vi "3D_Traverse_move.vi"(0 "Mode":T5=enum."Read traverse position", 1 "Position":sgl[](array[numeric])=[0.0, 0.0, 0.0] format="%#.2f", 2 "Extra command String":string, 3 "Work in Tunnel Coordinates":T3, 4 "Home":T2, 5 "Simulate/Run":T4=enum."Run VI", 6 "Route Checking?":bool=TRUE, 7 "Traverse name":string, 8 "Display Error":bool=TRUE, 9 "Backlash Compensation?":bool=TRUE, 10 "Row Number":i32=-1, 11 "Last Part of Move?":bool=TRUE, 13 "Currently on Point":i32=-1) -> (12 "Model:    Roll        Pitch         Yaw  (deg)":sgl[](array[numeric]) caption="ModelRollPitchYaw (deg)" format="%#.2f", 14 "Trav Position achieved":sgl[](array[numeric]) format="%#.2f", 17 "Valid Steps before Trav to Trav (Tun Cord)":sgl[][](array[numeric]), 19 "Error String":string)   [LabVIEW 2022 SP3]
uses:
  Trav_mode.ctl
  Controls/User_Specific_mode.ctl
  Controls/Tunnel_Coordinates.ctl
  Controls/Home.ctl
  Controls/Position Feedback System.ctl
  Route mapping/Route_Display_Mode.ctl
  ADAM Client/Sub VIs/ADAM Controls/Quick_local_ADAM_Table.ctl
  Controls/In_Range.ctl
  Globals/Trav_pos_global.vi
  Globals/Preference_global.vi
  Globals/Constants_global.vi
  Route mapping/Route_mapping_global.vi
  Globals/Extra_Commands_Global.vi
panel:
  out "Position Feedback System":T1
  out "Feedback Correction":sgl[](array[numeric]) format="%#.2f"
  out "Start Position":sgl[](array[numeric])
  out "Move Time (s)":sgl
  in  "Position Offset":sgl[](array[numeric])=[0.0, 0.0, 0.0] step=1 format="%#.2f"
  out "Traverses Available":string[](array[string])
  in  "Traverse":u16(ring) items=["A_Tunnel", "A_Tunnel_Turntable", "Pitch_Yaw", "Pitch_Traverse", "Dynamixel_Pitch"]
  # "X                Y                   Z"
  # "X                Y                   Z"
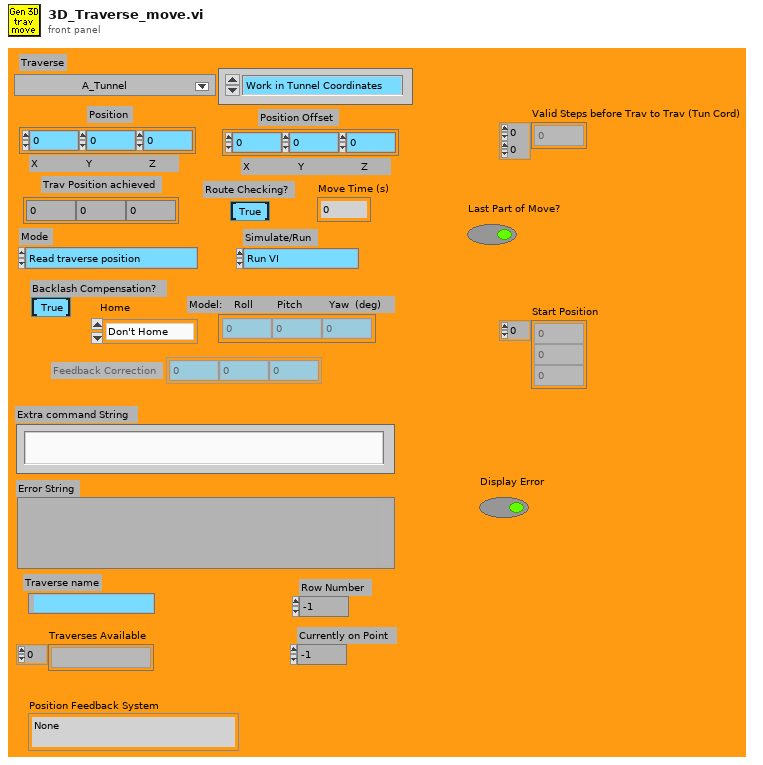
[diagram p1: front panel]
types:
  T1 = typedef "Position Feedback System.ctl" = enum16{"None", "OptiTrack"}
  T2 = typedef "Home.ctl" = enum16{"Don't Home", "Home  +X", "Home  -X", "Home  +Y", "Home  -Y", "Home  +Z", "Home  -Z"}
  T3 = typedef "Tunnel_Coordinates.ctl" = enum16{"Work in Tunnel Coordinates", "Work in Model Coordinates"}
  T4 = typedef "User_Specific_mode.ctl" = enum16{"Check VI only", "Run VI"}
  T5 = typedef "Trav_mode.ctl" = enum16{"Move traverse", "Read traverse position", "Teach Position"}
  T6 = enum8{"Enabled", "Disabled", "Disabled and Grayed Out"}
  T7 = enum16{"To Traverse Coordinates", "To User Coordinates"}
  T8 = typedef "Route_Display_Mode.ctl" = enum16{"Display View Always", "Display View on Crash"}
  T9 = typedef "Quick_local_ADAM_Table.ctl" = enum16{"Read Global", "Load Global From ADAM Table", "Write Global"}
  T10 = typedef "In_Range.ctl" = enum16{"%", "±", "% & ±"}
  T11 = typedef "Traverse_cluster.ctl" = cluster{"Start X":sgl, "Start Y":sgl, "Start Z":sgl, "End X":sgl, "End Y":sgl, "End Z":sgl, "nPoints":i32, "Spacing":T12, "Filename":path, "Tunnel Speed":dbl, "Averaging time (mins)":dbl, "Extra Commands":string, "Carrier_1 Q (l/min)":dbl, "Carrier_2 Q (l/min)":dbl, "Trace Gas Concentration (%)":dbl, "Specific Arguments":string, "Comments":string, "Row No":i32, "Row Type Selector":T13, "EstCompl":string, "Row Duration (mins)":dbl, "nValidPoints":i32, "Meas Setup File":string}
  T12 = typedef "Spacing.ctl" = enum16{"Linear", "Log", "Gauss", "Specified", "N/A"}
  T13 = typedef "Multi_run_mode.ctl" = enum16{"Move Traverse Only", "Set Tunnel Speed Only", "Set Source Only", "Set Measurement Conditions", "Single Measurement", "Vertical Profile", "Lateral Profile", "Longitudinal Profile", "Multi-Axis Profile", "Explore Volume", "Auto Calibrate", "Meas Fast FID Bkgnd", "Check Beam Power", "Scanning Valve Measurement", "Run VI Named:", "Set ADAM Ch", "Wait (minutes)", "Send Message", "Synchronize With:", "Fall Back to this Row", "Turn Off Row Repeating", "Traverse 3D Volume", "Blank Row", "Jump to Fall Back Row"}
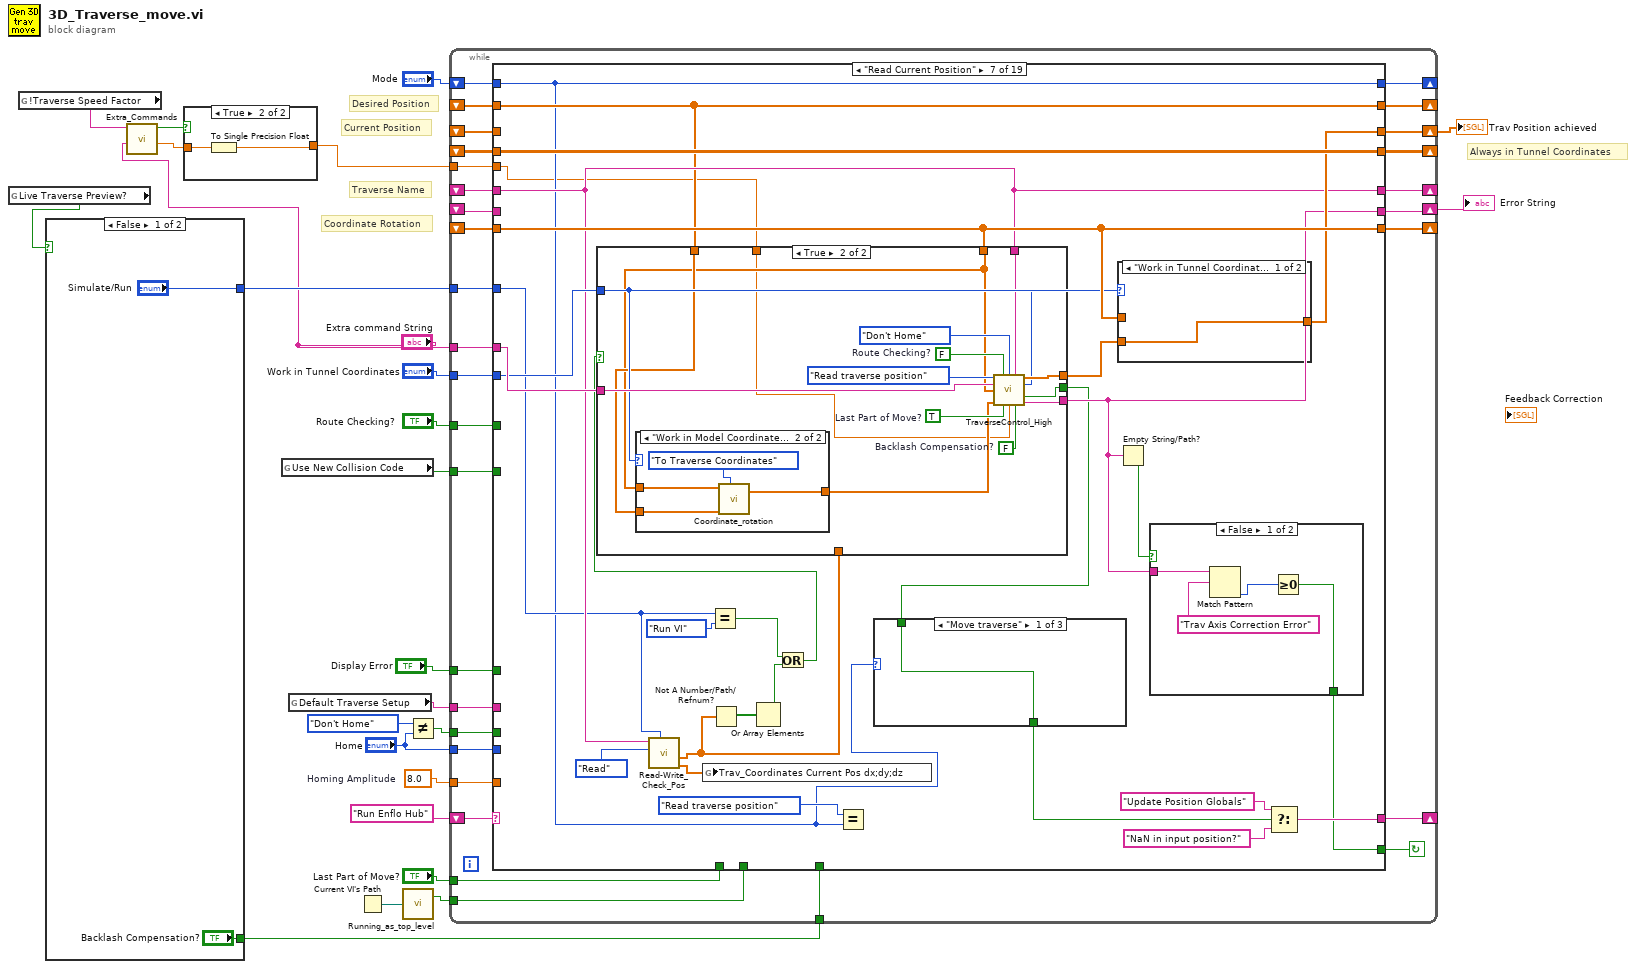
[diagram p0: block diagram]
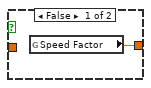
[diagram p2: hidden frame]
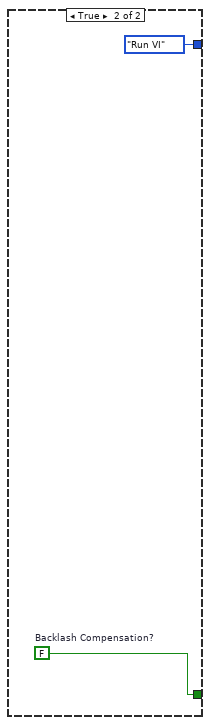
[diagram p3: hidden frame]
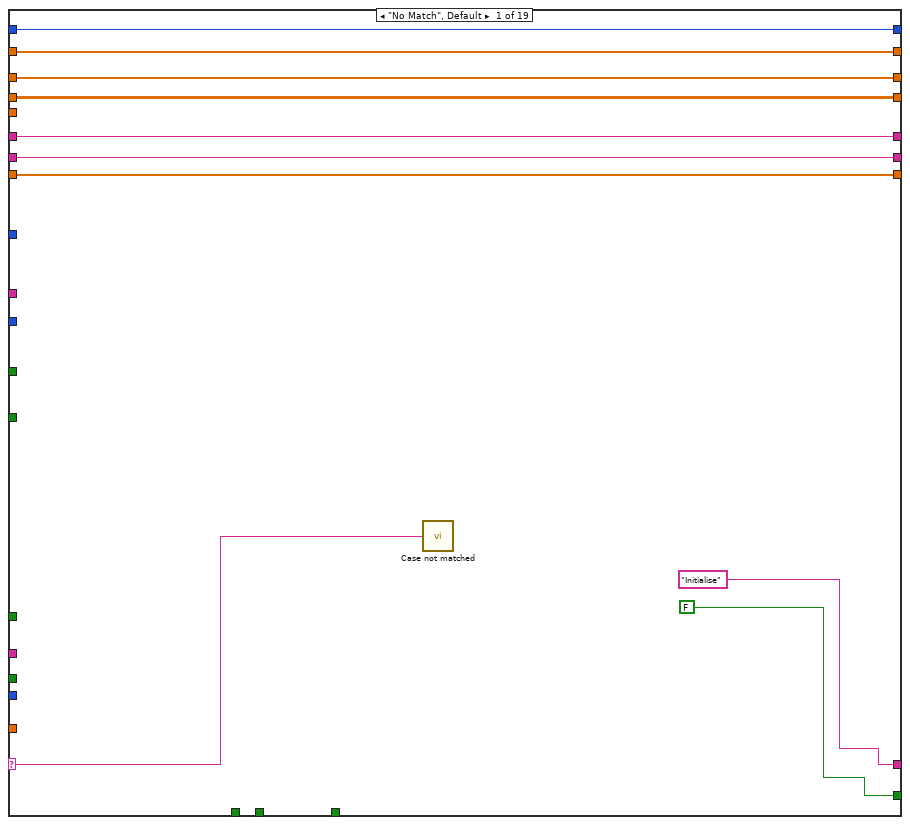
[diagram p4: hidden frame]
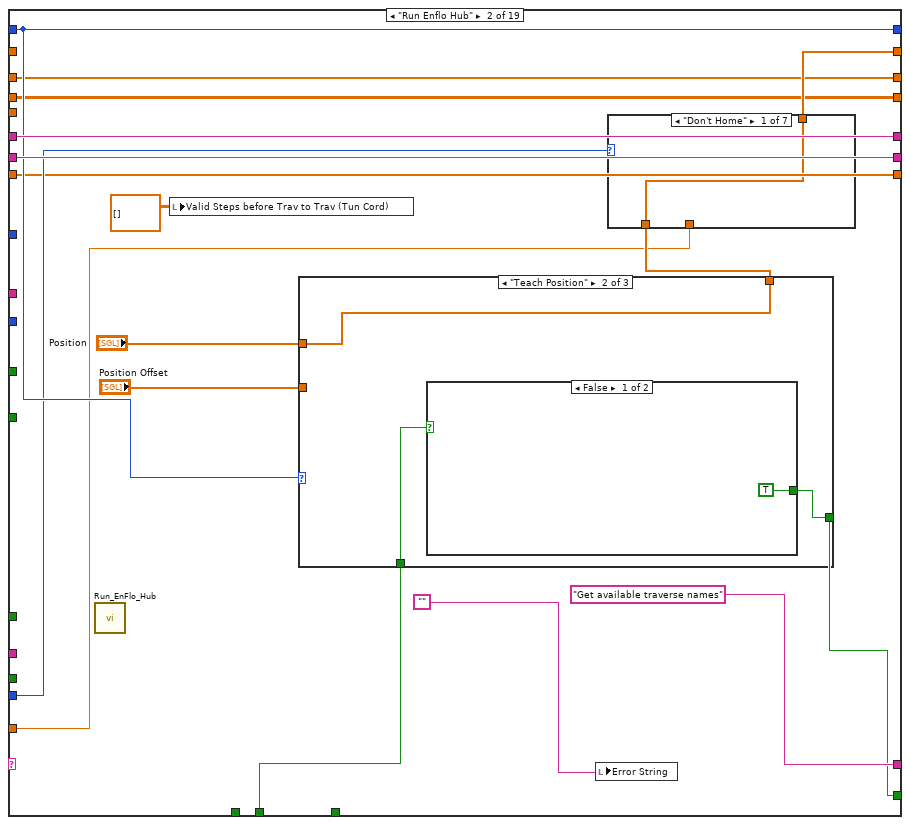
[diagram p5: hidden frame]
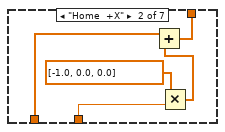
[diagram p6: hidden frame]
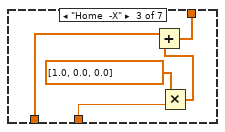
[diagram p7: hidden frame]
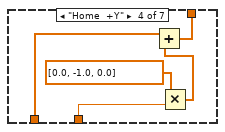
[diagram p8: hidden frame]
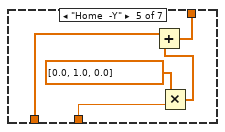
[diagram p9: hidden frame]
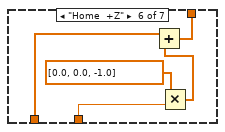
[diagram p10: hidden frame]
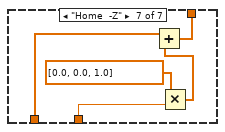
[diagram p11: hidden frame]
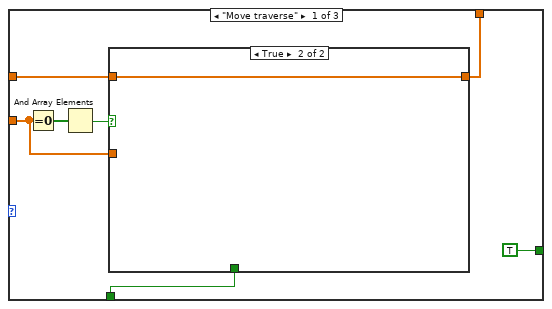
[diagram p12: hidden frame]
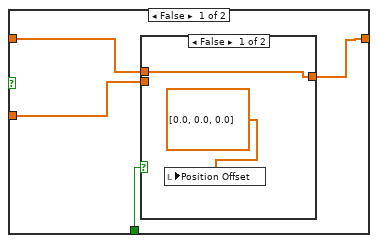
[diagram p13: hidden frame]
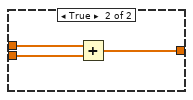
[diagram p14: hidden frame]
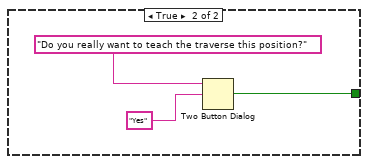
[diagram p15: hidden frame]
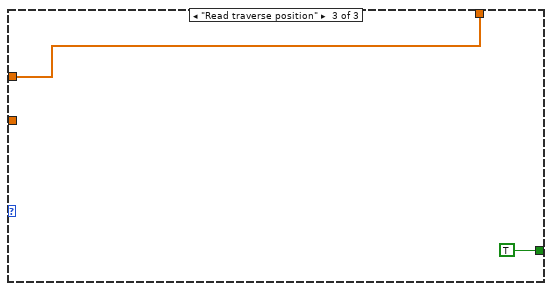
[diagram p16: hidden frame]
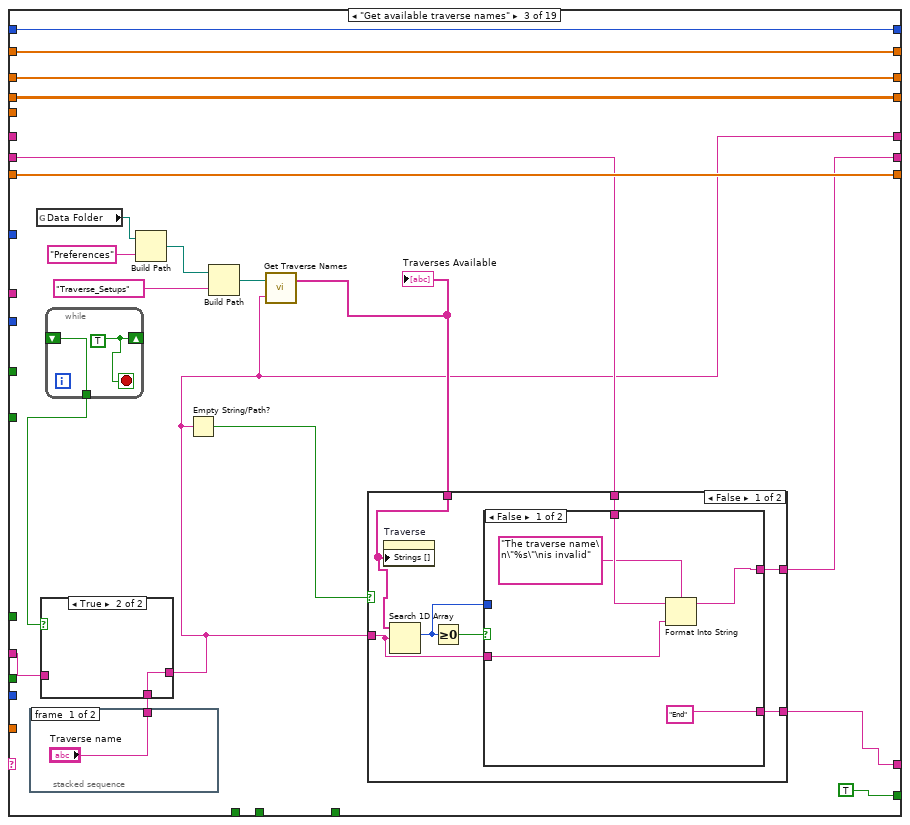
[diagram p17: hidden frame]
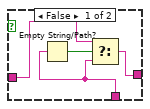
[diagram p18: hidden frame]
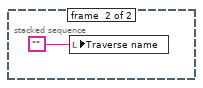
[diagram p19: hidden frame]
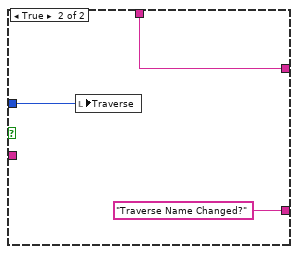
[diagram p20: hidden frame]
diagram:
  w16 = sgl 8.0  # Homing Amplitude
  # "Desired Position"
  # "Always in Tunnel Coordinates"
  # "Current Position"
  # "Coordinate Rotation"
  # "Traverse Name"
  n1 = global read "Trav_pos_global.vi" "Live Traverse Preview?"() -> (w6:bool)
  n2 = global read "Extra_Commands_Global.vi" "!Traverse Speed Factor"() -> (w5:string)
  n3 = case shown="False" w6 {
    tunnel: ["Simulate/Run" User_Specific_mode."Run VI" ("Simulate/Run")] -> w23
    tunnel: ["Backlash Compensation?" w27] -> w7
    frame False {
    }
    frame True {
      w27 = FALSE  # Backlash Compensation?
    }
  }
  n4 = call "Extra_Commands.vi"("String to Search"="Extra command String", "Command"=w5) -> ("Numeric Value"=w4:dbl, "Command Found"=w3:bool)  [unwired: 1 in, 3 out]
  n5 = case shown="True" w3 {
    tunnel: w4 -> [_ w31]
    tunnel: [w29 w30] -> w1
    frame False {
      n6 = global read "Trav_pos_global.vi" "Speed Factor"() -> (w29:sgl)
    }
    frame True {
      n7 = To Single Precision Float(number=w31) -> (single precision float=w30:sgl)
    }
  }
  n8 = global read "Preference_global.vi" "Use New Collision Code"() -> (w12:bool)
  n9 = global read "Trav_pos_global.vi" "Default Traverse Setup"() -> (w18:string)
  n10 = Current VI's Path() -> (path=w10:path)
  n11 = call "Running_as_top_level.vi"("Vi path name"=w10) -> ("Top Level"=w9:bool)  [unwired: 1 out]
  n12 = Not Equal?(x=Home."Don't Home" ("Home"), y="Home") -> (x != y?=w13:bool)
  n13 = while {
    shift-left: "Run Enflo Hub" -> [w60]
    shift-right: [w61] -> _
    shift-right: [w58] -> _
    shift-left: _ -> [w34]
    tunnel: w23 -> [w59]
    shift-right: [w57] -> w22
    shift-left: _ -> [w56]
    shift-right: [w54] -> _
    shift-left: _ -> [w55]
    shift-right: [w51] -> _
    shift-left: _ -> [w50]
    shift-right: [w52] -> w19
    shift-left: _ -> [w53]
    tunnel: "Work in Tunnel Coordinates" -> [w49]
    tunnel: "Route Checking?" -> [w48]
    tunnel: w18 -> [w47]
    shift-right: [w46] -> _
    shift-left: _ -> [w45]
    shift-right: [w43] -> _
    shift-left: "Mode" -> [w44]
    tunnel: "Home" -> [w42]
    tunnel: w16 -> [w41]
    tunnel: w13 -> [w40]
    tunnel: w12 -> [w39]
    tunnel: "Last Part of Move?" -> [w38]
    tunnel: w9 -> [w37]
    tunnel: "Extra command String" -> [w36]
    tunnel: "Display Error" -> [w35]
    tunnel: w7 -> [w33]
    tunnel: w1 -> [w32]
    stop <- w62 continue-if-true
    n14 = case shown="\"Read Current Position\"" w60 {
      selector: w60 -> [w63 _ _ _ _ _ _ _ _ _ _ _ _ _ _ _ _ _ _]
      tunnel: [FALSE w85 TRUE TRUE w220 TRUE w307 TRUE ("T button?") w400 w526 w636 TRUE ("Display Trav 2 Trav Error") TRUE ("Display Trav 2 Trav Error") TRUE ("Display Trav 2 Trav Error") TRUE ("Display Trav 2 Trav Error") TRUE TRUE TRUE FALSE] -> w62
      tunnel: ["Initialise" "Get available traverse names" w158 "Traverse Name Changed?" "Mode" w260 w312 w358 w401 w527 w637 w666 "End" w721 "Update Position Globals" "Update Position Globals" "Tidy up" "End" "End"] -> w61
      tunnel: w59 -> [_ _ _ _ w214 w261 w296 _ w412 w537 w640 _ _ w732 _ _ w856 w898 w989]
      tunnel: [w70 w88 w147 w193 w226 w257 w304 w369 w404 w530 w634 w677 w705 w738 w765 w800 w855 w903 w993] -> w58
      tunnel: [w69 w87 w157 w205 w221 w262 w308 w366 w394 w539 w630 w661 w710 w735 w777 w787 w859 w905 w995] -> w57
      tunnel: w34 -> [w70 w88 _ _ w226 w257 w304 w369 w404 w530 w634 w677 w705 w738 w765 w800 w855 w903 w993]
      tunnel: w56 -> [w69 w87 w156 w205 _ w262 _ w366 _ _ w625 w673 w710 w735 w777 _ w859 w906 w994]
      tunnel: w55 -> [w68 w76 w166 w204 _ w254 w317 w356 w405 w531 w633 w669 w708 w741 w771 w799 w852 w908 w999]
      tunnel: [w68 w76 w166 w204 w225 w254 w317 w356 w405 w531 w633 w669 w708 w741 w771 w799 w852 w908 w999] -> w54
      tunnel: w53 -> [w67 w75 w165 w203 w235 w253 _ w355 w413 w538 w626 w676 w714 w740 w770 _ w854 w907 w1000]
      tunnel: [w67 w75 w165 w203 w235 w253 w311 w355 w413 w538 w628 w676 w714 w740 w770 w797 w854 w907 w1000] -> w52
      tunnel: [w66 w74 w164 w202 w227 w251 w318 w360 w403 w529 w623 w675 w713 w739 w769 w791 w860 w909 w1004] -> w51
      tunnel: w50 -> [w66 w74 w164 w202 w227 w250 w318 w359 _ _ w623 w675 w713 w739 w769 w791 w860 w909 w1004]
      tunnel: w49 -> [_ _ _ _ _ w255 w306 w357 w414 w540 w632 w670 w709 _ w772 w782 w853 _ w1001]
      tunnel: w48 -> [_ _ _ _ _ _ _ w362 _ _ _ _ _ _ _ w795 _ _ _]
      tunnel: w47 -> [_ _ w151 w197 _ _ _ _ _ _ _ _ _ _ _ _ _ _ _]
      tunnel: [w65 w80 w154 w195 w228 w252 w295 w361 w411 w536 w627 w672 w707 w727 w776 w794 w858 w902 w1002] -> w46
      tunnel: w45 -> [w65 _ w154 w195 w228 w252 w295 w363 w411 w536 w627 w672 w707 w727 w776 w794 w858 w902 w1002]
      tunnel: w44 -> [w64 w82 w153 w194 w231 w256 w294 w367 w410 w535 w641 w671 w715 w726 w775 w793 w857 w901 w997]
      tunnel: [w64 w82 w153 w194 w232 w256 w294 w367 w410 w535 w641 w671 w715 w726 w775 w793 w857 w901 w997] -> w43
      tunnel: w42 -> [_ w79 _ _ _ _ _ _ w409 w534 _ _ _ _ _ w788 _ w900 _]
      tunnel: w41 -> [_ w78 _ _ _ _ _ _ w407 w532 _ _ _ _ _ _ _ w899 _]
      tunnel: w40 -> [_ _ _ _ _ _ _ _ _ _ _ _ _ _ _ _ _ w897 _]
      tunnel: w39 -> [_ _ _ _ w229 _ _ _ w406 _ _ w660 _ _ _ _ _ _ _]
      tunnel: w38 -> [_ _ _ _ _ _ _ _ _ _ _ _ _ _ _ w783 _ _ _]
      tunnel: w37 -> [_ w77 _ _ w224 _ _ _ _ _ _ w668 _ _ _ w786 _ _ _]
      tunnel: w36 -> [_ _ _ _ _ _ w310 _ _ _ _ _ _ _ _ w779 _ _ _]
      tunnel: w35 -> [_ _ _ _ _ _ _ _ w399 w525 w635 _ _ _ _ _ _ _ _]
      tunnel: w33 -> [_ _ _ _ _ _ _ _ _ _ _ _ _ _ w766 w780 _ _ _]
      tunnel: w32 -> [_ _ _ _ _ _ w291 _ _ _ _ _ _ _ _ w778 _ _ _]
      frame "No Match", Default {
        n15 = call "Case not matched.vi"("Case Name not Matched"=w63) -> ()
      }
      frame "Run Enflo Hub" {
        n16 = call "Run_EnFlo_Hub.vi"() -> ()  [unwired: 1 in, 7 out]
        n17 = local write "Valid Steps before Trav to Trav (Tun Cord)"(sgl[][] [] ("Valid Steps before Trav to Trav (Tun Cord)")) -> ()
        n18 = case shown="\"Teach Position\"" w82 {
          tunnel: [TRUE ("T button?") w140 TRUE ("T button?")] -> w85
          tunnel: [w124 w139 w146] -> w81
          tunnel: "Position" -> [w123 w139 w146]
          tunnel: "Position Offset" -> [w122 _ _]
          tunnel: w77 -> [w121 w138 _]
          frame "Move traverse" {
            n19 = Equal To 0?(x=w122) -> (x = 0?=w126:bool[])
            n20 = And Array Elements(Boolean array=w126) -> (logical AND=w125:bool)
            n21 = case shown="True" w125 {
              tunnel: [w129 w137] -> w124
              tunnel: w123 -> [w131 w137]
              tunnel: w122 -> [w130 _]
              tunnel: w121 -> [w128 _]
              frame False {
                n22 = case shown="False" w128 {
                  tunnel: w131 -> [w133 w136]
                  tunnel: w130 -> [_ w135]
                  tunnel: [w133 w134] -> w129
                  frame False {
                    n23 = local write "Position Offset"(sgl[] [0.0, 0.0, 0.0] ("Position Increment")) -> ()
                  }
                  frame True {
                    n24 = Add(x=w136, y=w135) -> (x+y=w134:sgl[])
                  }
                }
              }
              frame True {
              }
            }
          }
          frame "Teach Position" {
            n25 = case shown="False" w138 {
              tunnel: [TRUE ("T button?") w142] -> w140
              frame False {
              }
              frame True {
                n26 = Two Button Dialog(message="Do you really want to teach the traverse this position?", 2:"Yes" ("T button name (\"OK\")")) -> (T button?=w142:bool)  [unwired: 1 out]
              }
            }
          }
          frame "Read traverse position" {
          }
        }
        n27 = local write "Error String"("") -> ()
        n28 = case shown="\"Don't Home\"" w79 {
          tunnel: [w90 w94 w99 w104 w109 w114 w119] -> w80
          tunnel: w81 -> [w90 w95 w100 w105 w110 w115 w120]
          tunnel: w78 -> [_ w91 w96 w101 w106 w111 w116]
          frame "Don't Home" {
          }
          frame "Home  +X" {
            n29 = Multiply(x=sgl[] [-1.0, 0.0, 0.0] ("y"), y=w91) -> (x*y=w92:sgl[])
            n30 = Add(x=w95, y=w92) -> (x+y=w94:sgl[])
          }
          frame "Home  -X" {
            n31 = Multiply(x=sgl[] [1.0, 0.0, 0.0] ("y"), y=w96) -> (x*y=w97:sgl[])
            n32 = Add(x=w100, y=w97) -> (x+y=w99:sgl[])
          }
          frame "Home  +Y" {
            n33 = Multiply(x=sgl[] [0.0, -1.0, 0.0] ("y"), y=w101) -> (x*y=w102:sgl[])
            n34 = Add(x=w105, y=w102) -> (x+y=w104:sgl[])
          }
          frame "Home  -Y" {
            n35 = Multiply(x=sgl[] [0.0, 1.0, 0.0] ("y"), y=w106) -> (x*y=w107:sgl[])
            n36 = Add(x=w110, y=w107) -> (x+y=w109:sgl[])
          }
          frame "Home  +Z" {
            n37 = Multiply(x=sgl[] [0.0, 0.0, -1.0] ("y"), y=w111) -> (x*y=w112:sgl[])
            n38 = Add(x=w115, y=w112) -> (x+y=w114:sgl[])
          }
          frame "Home  -Z" {
            n39 = Multiply(x=sgl[] [0.0, 0.0, 1.0] ("y"), y=w116) -> (x*y=w117:sgl[])
            n40 = Add(x=w120, y=w117) -> (x+y=w119:sgl[])
          }
        }
      }
      frame "Get available traverse names" {
        n41 = stacked-sequence {
          tunnel: ["Traverse name" _] -> w150
          frame #0 {
          }
          frame #1 {
            n42 = local write "Traverse name"("") -> ()
          }
        }
        n43 = global read "Constants_global.vi" "Data Folder"() -> (w161:path)
        n44 = while {
          shift-right: [w174] -> _
          shift-left: _ -> [w175]
          tunnel: [w175] -> w152
          stop <- w174 stop-if-true
          w174 = TRUE
        }
        n45 = case shown="True" w152 {
          tunnel: [w169 w171] -> w147
          tunnel: w151 -> [w168 _]
          tunnel: w150 -> [w167 w171]
          frame False {
            n46 = Empty String/Path?(string/path=w167) -> (empty?=w170:bool)
            n47 = Select(t=w168, s=w170, f=w167) -> (s? t:f=w169:string)
          }
          frame True {
          }
        }
        n48 = Build Path(base path=w161, name or relative path="Preferences") -> (appended path=w163:path)
        n49 = Empty String/Path?(string/path=w147) -> (empty?=w159:bool)
        n50 = Build Path(base path=w163, name or relative path="Traverse_Setups") -> (appended path=w149:path)
        n51 = call "Get Traverse Names.vi"("Traverse name"=w147, "Traverse\nSetup\nFolder"=w149) -> ("Traverse Names"=w148:string[])  [unwired: 1 out]
        "Traverses Available" <- w148
        n52 = case shown="False" w159 {
          tunnel: [w179 "Read menu ring"] -> w158
          tunnel: w148 -> [w176 _]
          tunnel: w147 -> [w182 _]
          tunnel: [w181 w191] -> w157
          tunnel: w156 -> [w180 w191]
          frame False {
            n53 = property on="Traverse" class="Ring (strict)"("Strings []"=w176) -> ()  [unwired: 2 in, 2 out]
            n54 = Search 1D Array(1D array=w176, element=w182) -> (index of element=w177:i32)  [unwired: 1 out]
            n55 = Greater Or Equal To 0?(x=w177) -> (x >= 0?=w178:bool)
            n56 = case shown="False" w178 {
              tunnel: w182 -> [w187 _]
              tunnel: [w184 w190] -> w181
              tunnel: w180 -> [w186 w190]
              tunnel: ["End" "Traverse Name Changed?"] -> w179
              tunnel: w177 -> [_ w188]
              frame False {
                n57 = Format Into String(format string="The traverse name\n\"%s\"\nis invalid", initial string=w186, w187) -> (resulting string=w184:string)  [unwired: 1 in, 1 out]
              }
              frame True {
                n58 = local write "Traverse"(w188) -> ()
              }
            }
          }
          frame True {
          }
        }
      }
      frame "Read menu ring" {
        n59 = local read "Traverses Available"() -> (w198:string[])
        n60 = property on="Traverse" class="Ring (strict)"() -> ("Strings []"=w201:string[])  [unwired: 2 in, 2 out]
        n61 = Index Array(array=w201, index="Traverse") -> (element=w196:string)
        n62 = Search 1D Array(1D array=w198, element=w196) -> (index of element=w199:i32)  [unwired: 1 out]
        n63 = case shown="-1" w199 {
          tunnel: w198 -> [_ w211]
          tunnel: w197 -> [_ w209]
          tunnel: [w208 w209] -> w193
          tunnel: w196 -> [w208 _]
          frame 0, Default {
          }
          frame -1 {
            n64 = property on="Traverse" class="Ring (strict)"("Strings []"=w211) -> ()  [unwired: 2 in, 2 out]
            n65 = Search 1D Array(1D array=w211, element=w209) -> (index of element=w210:i32)  [unwired: 1 out]
            n66 = local write "Traverse"(w210) -> ()
          }
        }
      }
      frame "Traverse Name Changed?" {
        n67 = Select(t=User_Specific_mode."Run VI", s=w224, f=w214) -> (s? t:f=w222:T4)
        n68 = call "Get Model Roll Pitch Yaw.vi"("Traverse Name"=w226, "Mode"=w222) -> ("Model:    Roll        Pitch         Yaw  (deg)"=w225:sgl[], "Position Feedback System"=w213:T1, "Error String"=w221:string)
        "Model:    Roll        Pitch         Yaw  (deg)" <- w225
        "Position Feedback System" <- w213
        n69 = case shown="\"OptiTrack\"" w213 {
          tunnel: [T6."Disabled and Grayed Out" ("Disabled") T6."Disabled" ("Disabled")] -> w212
          frame "None" {
          }
          frame "OptiTrack" {
          }
        }
        n70 = global read "Route_mapping_global.vi" "Traverse Setup"() -> (w230:string)
        n71 = Empty String/Path?(string/path=w221) -> (empty?=w220:bool)
        n72 = global read "Trav_pos_global.vi" "Mirror Up?"() -> (w219:bool)
        n73 = property on="Feedback Correction" class="Arr (strict)"("DisabledEnum"=w212) -> ()  [unwired: 2 in, 2 out]
        n74 = feedback-in #1(w219) -> ()
        n75 = feedback #1() -> (w218:bool)  [unwired: 1 in]
        n76 = Equal?(x=w219, y=w218) -> (x = y?=w216:bool)
        n77 = Equal?(x=w230, y=w226) -> (x = y?=w217:bool)
        n78 = And(x=w216, y=w217) -> (x .and. y?=w215:bool)
        n79 = case shown="False" w215 {
          tunnel: w226 -> [w242 _]
          tunnel: [w240 FALSE ("Top Level")] -> w234
          tunnel: w229 -> [w241 _]
          tunnel: w224 -> [w240 _]
          tunnel: w214 -> [w239 _]
          frame False {
            n80 = case shown="False" w241 {
              tunnel: w242 -> [w244 w247]
              tunnel: w239 -> [w243 w246]
              frame False {
                w245 = FALSE  # Show Panel?
                n81 = call "Traverse_Space.vi"("Simulate/Run"=w243, "Show Panel?"=w245, "Traverse Setup"=w244) -> ()  [unwired: 1 in, 7 out]
              }
              frame True {
                w248 = FALSE  # Show Panel?
                n82 = call "Traverse_Space_for new collision code.vi"("Simulate/Run"=w246, "Show Panel?"=w248, "Traverse Setup"=w247) -> ()  [unwired: 7 in, 1 out]
              }
            }
          }
          frame True {
          }
        }
        n83 = Select(t=Trav_mode."Read traverse position" ("Mode"), s=w234, f=w231) -> (s? t:f=w232:T5)
      }
      frame "Mode" {
        n84 = case shown="\"Run VI\"" w261 {
          tunnel: w256 -> [_ w274]
          tunnel: [w265 w273] -> w260
          tunnel: "Execute case" -> [_ w272]
          tunnel: "Read Current Position" -> [w265 w271]
          tunnel: w255 -> [_ w270]
          tunnel: w254 -> [_ w269]
          tunnel: w252 -> [_ w268]
          tunnel: [w264 w267] -> w251
          tunnel: w250 -> [w264 w266]
          frame "Check VI only" {
          }
          frame "Run VI" {
            n85 = case shown="\"Teach Position\"" w274 {
              tunnel: [w275 w279 w285] -> w273
              tunnel: w272 -> [_ w279 w285]
              tunnel: w271 -> [w275 _ _]
              tunnel: w270 -> [_ _ w284]
              tunnel: w269 -> [_ _ w283]
              tunnel: w268 -> [_ _ w282]
              tunnel: [w276 w277 w280] -> w267
              tunnel: w266 -> [w276 _ _]
              frame "Move traverse" {
              }
              frame "Read traverse position" {
                n86 = Build Array(sgl[] [0.0, 0.0, 0.0] ("Output Position")) -> (w277:sgl[][])
              }
              frame "Teach Position" {
                n87 = case shown="\"Work in Model Coordinates\"" w284 {
                  tunnel: [w286 w289] -> w281
                  tunnel: w283 -> [_ w288]
                  tunnel: w282 -> [w286 w287]
                  frame "Work in Tunnel Coordinates" {
                  }
                  frame "Work in Model Coordinates" {
                    n88 = call "Coordinate_rotation.vi"("Roll-Pitch-Yaw"=w288, "Input Position"=w287, "Mode"=T7."To Traverse Coordinates") -> ("Output Position"=w289:sgl[])  [unwired: 2 in, 1 out]
                  }
                }
                n89 = Build Array(w281) -> (w280:sgl[][])
              }
            }
          }
        }
      }
      frame "Read Current Position" {
        n90 = call "Read-Write_Check_Pos.vi"("Simulate/Run"=w296, "Mode"=enum16{"Read", "Write"}."Read", "Traverse Name"=w304) -> ("!Offset Position by dx;dy;dz  Output"=w303:sgl[], "Position Output"=w302:sgl[])  [unwired: 4 in, 1 out]
        n91 = global write "Trav_pos_global.vi" "Trav_Coordinates Current Pos dx;dy;dz"(w303) -> ()
        n92 = Equal?(x=w296, y=User_Specific_mode."Run VI" ("Simulate/Run")) -> (x = y?=w299:bool)
        n93 = Not A Number/Path/Refnum?(number/path/refnum=w302) -> (NaN/Path/Refnum?=w301:bool[])
        n94 = Or Array Elements(Boolean array=w301) -> (logical OR=w298:bool)
        n95 = Or(x=w299, y=w298) -> (x .or. y?=w297:bool)
        n96 = case shown="True" w297 {
          tunnel: w304 -> [_ w343]
          tunnel: ["" w336] -> w308
          tunnel: w317 -> [_ w332]
          tunnel: [w328 w344] -> w316
          tunnel: w295 -> [_ w334]
          tunnel: w310 -> [_ w337]
          tunnel: w306 -> [_ w335]
          tunnel: w302 -> [w328 _]
          tunnel: [FALSE ("Position Correct") w331] -> w293
          tunnel: w291 -> [_ w330]
          frame False {
          }
          frame True {
            w339 = TRUE  # Last Part of Move?
            w342 = FALSE  # Route Checking?
            w341 = FALSE  # Backlash Compensation?
            n97 = case shown="\"Work in Model Coordinates\"" w335 {
              tunnel: w334 -> [w345 w347]
              tunnel: [w345 w348] -> w333
              tunnel: w332 -> [_ w346]
              frame "Work in Tunnel Coordinates" {
              }
              frame "Work in Model Coordinates" {
                n98 = call "Coordinate_rotation.vi"("Roll-Pitch-Yaw"=w346, "Input Position"=w347, "Mode"=T7."To Traverse Coordinates") -> ("Output Position"=w348:sgl[])  [unwired: 2 in, 1 out]
              }
            }
            n99 = call "TraverseControl_High.vi"("Mode"=Trav_mode."Read traverse position", "Route Checking?"=w342, "Home"=Home."Don't Home", "Traverse Name"=w343, "Extra command String"=w337, "Work in Tunnel Coordinates"=w335, "Model       Roll      Pitch       Yaw (deg)"=w332, "Position input XYZ Always Tunnel"=w333, "Last Part of Move?"=w339, "Speed Factor"=w330, "Backlash Compensation?"=w341) -> ("Position Output XYZ"=w344:sgl[], "Position Correct"=w331:bool, "Error String"=w336:string)  [unwired: 2 in]
          }
        }
        n100 = Equal?(x=Trav_mode."Read traverse position" ("Mode"), y=w294) -> ()  [unwired: 1 out]
        n101 = case shown="\"Move traverse\"" w294 {
          tunnel: [w319 TRUE FALSE] -> w292
          tunnel: w293 -> [w319 _ _]
          frame "Move traverse" {
          }
          frame "Read traverse position" {
          }
          frame "Teach Position" {
          }
        }
        n102 = case shown="\"Work in Tunnel Coordinates\"" w306 {
          tunnel: w316 -> [w350 w352]
          tunnel: [w350 w353] -> w311
          tunnel: w317 -> [_ w351]
          frame "Work in Tunnel Coordinates" {
          }
          frame "Work in Model Coordinates" {
            n103 = call "Coordinate_rotation.vi"("Roll-Pitch-Yaw"=w351, "Input Position"=w352, "Mode"=T7."To User Coordinates") -> ("Output Position"=w353:sgl[])  [unwired: 2 in, 1 out]
          }
        }
        n104 = Empty String/Path?(string/path=w308) -> (empty?=w309:bool)
        n105 = case shown="False" w309 {
          tunnel: w308 -> [w324 _]
          tunnel: [w322 TRUE] -> w307
          frame False {
            n106 = Match Pattern(string=w324, regular expression="Trav Axis Correction Error" ("string")) -> (offset past match=w323:i32)  [unwired: 4 out]
            n107 = Greater Or Equal To 0?(x=w323) -> (x >= 0?=w322:bool)
          }
          frame True {
          }
        }
        n108 = Select(t="Update Position Globals", s=w292, f="NaN in input position?") -> (s? t:f=w312:string)
      }
      frame "NaN in input position?" {
        n109 = Not A Number/Path/Refnum?(number/path/refnum=w363) -> (NaN/Path/Refnum?=w365:bool[])
        n110 = Or Array Elements(Boolean array=w365) -> (logical OR=w364:bool)
        n111 = case shown="True" w364 {
          tunnel: w365 -> [_ w387]
          tunnel: w355 -> [_ w386]
          tunnel: w363 -> [w383 w385]
          tunnel: [w383 w384] -> w361
          frame False {
          }
          frame True {
            n112 = for {
              tunnel: w387 -> [w391] mode=indexing
              tunnel: w386 -> [w390] mode=indexing
              tunnel: [w389] -> w384 mode=indexing
              tunnel: w385 -> [w388] mode=indexing
              n113 = case shown="True" w391 {
                tunnel: w390 -> [_ w393]
                tunnel: [w392 w393] -> w389
                tunnel: w388 -> [w392 _]
                frame False {
                }
                frame True {
                }
              }
            }
            n114 = local write "Position"(w384) -> ()
          }
        }
        n115 = case shown="True" w362 {
          tunnel: w361 -> [w370 _]
          tunnel: [w375 w382] -> w360
          tunnel: w359 -> [_ w382]
          tunnel: ["Execute case" "Perform Route Check"] -> w358
          tunnel: w357 -> [w373 _]
          tunnel: w356 -> [w371 _]
          frame False {
            n116 = case shown="\"Work in Model Coordinates\"" w373 {
              tunnel: [w376 w379] -> w372
              tunnel: w371 -> [_ w378]
              tunnel: w370 -> [w376 w377]
              frame "Work in Tunnel Coordinates" {
              }
              frame "Work in Model Coordinates" {
                n117 = call "Coordinate_rotation.vi"("Roll-Pitch-Yaw"=w378, "Input Position"=w377, "Mode"=T7."To Traverse Coordinates") -> ("Output Position"=w379:sgl[])  [unwired: 2 in, 1 out]
              }
            }
            n118 = Build Array(w372) -> (w375:sgl[][])
          }
          frame True {
          }
        }
        "Start Position" <- w355
      }
      frame "Perform Route Check" {
        n119 = case shown="True" w406 {
          tunnel: w414 -> [w436 w457]
          tunnel: [w425 w446] -> w395
          tunnel: w413 -> [w435 w455]
          tunnel: w412 -> [w427 w454]
          tunnel: w404 -> [w428 w453]
          tunnel: w411 -> [w434 w452]
          tunnel: [w430 w448] -> w408
          tunnel: w405 -> [w429 w450]
          tunnel: [w419 w445] -> w398
          tunnel: "Route Error" -> [w421 w445]
          frame True {
            w423 = "Invalid Destination point "
            n120 = case shown="\"Work in Tunnel Coordinates\"" w436 {
              tunnel: w429 -> [_ w443]
              tunnel: w434 -> [w437 w439]
              tunnel: w435 -> [w438 w442]
              tunnel: [w437 w441] -> w433
              tunnel: [w438 w440] -> w431
              frame "Work in Tunnel Coordinates" {
              }
              frame "Work in Model Coordinates" {
                w444 = T7."To Traverse Coordinates" ("Mode")
                n121 = call "Coordinate_rotation.vi"("Roll-Pitch-Yaw"=w443, "Input Position"=w442, "Mode"=w444) -> ("Output Position"=w440:sgl[])  [unwired: 2 in, 1 out]
                n122 = call "Coordinate_rotation.vi"("Roll-Pitch-Yaw"=w443, "Input Position"=w439, "Mode"=w444) -> ("Output Position"=w441:sgl[])  [unwired: 2 in, 1 out]
              }
            }
            n123 = call "Check_with_Jump_PN.vi"("Current position"=w431, "Traverse Name"=w428, "Simulate/Run"=w427, "New Position"=w433, "Traverse Active Parts"=cluster{"X":bool, "XY":bool, "XYZ":bool} {"X"=FALSE, "XY"=TRUE, "XYZ"=TRUE}, "Model       Roll      Pitch       Yaw (deg)"=w429) -> ("Error Comments"=w425:string, "Steps"=w430:sgl[][])  [unwired: 8 in]
            n124 = String Length(string=w423) -> (length=w426:i32)
            n125 = String Subset(string=w425, length (rest)=w426) -> (substring=w424:string)  [unwired: 1 in]
            n126 = Equal?(x=w424, y=w423) -> (x = y?=w422:bool)
            n127 = Select(t=w421, s=w422, f="Perform Route Check2") -> (s? t:f=w419:string)
          }
          frame False {
            n128 = case shown="\"Work in Tunnel Coordinates\"" w457 {
              tunnel: w450 -> [w466 _]
              tunnel: w452 -> [w462 w468]
              tunnel: w455 -> [w465 w469]
              tunnel: [w464 w468] -> w451
              tunnel: [w463 w469] -> w456
              frame "Work in Tunnel Coordinates" {
                w467 = T7."To User Coordinates" ("Mode")
                n129 = call "Coordinate_rotation.vi"("Roll-Pitch-Yaw"=w466, "Input Position"=w465, "Mode"=w467) -> ("Output Position"=w463:sgl[])  [unwired: 2 in, 1 out]
                n130 = call "Coordinate_rotation.vi"("Roll-Pitch-Yaw"=w466, "Input Position"=w462, "Mode"=w467) -> ("Output Position"=w464:sgl[])  [unwired: 2 in, 1 out]
              }
              frame "Work in Model Coordinates" {
              }
            }
            n131 = call "Check_with_Jump.vi"("Current position"=w456, "Traverse Name"=w453, "Simulate/Run"=w454, "New Position"=w451, "Model       Roll      Pitch       Yaw (deg)"=w450) -> ("Error Comments"=w446:string, "Steps"=w449:sgl[][])  [unwired: 9 in]
            n132 = for {
              tunnel: w450 -> [w461]
              tunnel: w449 -> [w460] mode=indexing
              tunnel: [w459] -> w448 mode=indexing
              tunnel: T7."To Traverse Coordinates" ("Mode") -> [w458]
              n133 = call "Coordinate_rotation.vi"("Roll-Pitch-Yaw"=w461, "Input Position"=w460, "Mode"=w458) -> ("Output Position"=w459:sgl[])  [unwired: 2 in, 1 out]
            }
          }
        }
        n134 = call "Load_Traverse_Configurations.vi"("Traverse Name"=w404) -> ("Error String"=w396:string)  [unwired: 10 in]
        n135 = Concatenate Strings(w396, w395) -> (w394:string)
        n136 = Empty String/Path?(string/path=w395) -> (empty?=w402:bool)
        n137 = case shown="\"Don't Home\"" w409 {
          tunnel: w408 -> [w470 w477 w485 w493 w501 w509 w517]
          tunnel: [w470 w476 w484 w492 w500 w508 w516] -> w403
          tunnel: w407 -> [_ w471 w479 w487 w495 w503 w511]
          frame "Don't Home" {
          }
          frame "Home  +X" {
            n138 = for {
              tunnel: [w478] -> w475
              tunnel: w477 -> [w478] mode=indexing
            }
            n139 = Multiply(x=sgl[] [2.0, 0.0, 0.0] ("y"), y=w471) -> (x*y=w472:sgl[])
            n140 = Add(x=w475, y=w472) -> (x+y=w474:sgl[])
            n141 = Build Array (concatenate)(w477, w474) -> (w476:sgl[][])
          }
          frame "Home  -X" {
            n142 = for {
              tunnel: [w486] -> w483
              tunnel: w485 -> [w486] mode=indexing
            }
            n143 = Multiply(x=sgl[] [-2.0, 0.0, 0.0] ("y"), y=w479) -> (x*y=w480:sgl[])
            n144 = Add(x=w483, y=w480) -> (x+y=w482:sgl[])
            n145 = Build Array (concatenate)(w485, w482) -> (w484:sgl[][])
          }
          frame "Home  +Y" {
            n146 = for {
              tunnel: [w494] -> w491
              tunnel: w493 -> [w494] mode=indexing
            }
            n147 = Multiply(x=sgl[] [0.0, 2.0, 0.0] ("y"), y=w487) -> (x*y=w488:sgl[])
            n148 = Add(x=w491, y=w488) -> (x+y=w490:sgl[])
            n149 = Build Array (concatenate)(w493, w490) -> (w492:sgl[][])
          }
          frame "Home  -Y" {
            n150 = for {
              tunnel: [w502] -> w499
              tunnel: w501 -> [w502] mode=indexing
            }
            n151 = Multiply(x=sgl[] [0.0, -2.0, 0.0] ("y"), y=w495) -> (x*y=w496:sgl[])
            n152 = Add(x=w499, y=w496) -> (x+y=w498:sgl[])
            n153 = Build Array (concatenate)(w501, w498) -> (w500:sgl[][])
          }
          frame "Home  +Z" {
            n154 = for {
              tunnel: [w510] -> w507
              tunnel: w509 -> [w510] mode=indexing
            }
            n155 = Multiply(x=sgl[] [0.0, 0.0, 2.0] ("y"), y=w503) -> (x*y=w504:sgl[])
            n156 = Add(x=w507, y=w504) -> (x+y=w506:sgl[])
            n157 = Build Array (concatenate)(w509, w506) -> (w508:sgl[][])
          }
          frame "Home  -Z" {
            n158 = for {
              tunnel: [w518] -> w515
              tunnel: w517 -> [w518] mode=indexing
            }
            n159 = Multiply(x=sgl[] [0.0, 0.0, -2.0] ("y"), y=w511) -> (x*y=w512:sgl[])
            n160 = Add(x=w515, y=w512) -> (x+y=w514:sgl[])
            n161 = Build Array (concatenate)(w517, w514) -> (w516:sgl[][])
          }
        }
        n162 = case shown="False" w402 {
          tunnel: [w415 "Perform Trav 2 Trav Check"] -> w401
          tunnel: [w416 TRUE] -> w400
          tunnel: w399 -> [w416 _]
          tunnel: w398 -> [w415 _]
          frame False {
          }
          frame True {
          }
        }
      }
      frame "Perform Route Check2" {
        # "New Collision Code Only"
        n163 = case shown="\"Work in Model Coordinates\"" w540 {
          tunnel: w531 -> [_ w568]
          tunnel: w536 -> [w562 w564]
          tunnel: w538 -> [w563 w567]
          tunnel: [w562 w566] -> w524
          tunnel: [w563 w565] -> w522
          frame "Work in Tunnel Coordinates" {
          }
          frame "Work in Model Coordinates" {
            w569 = T7."To Traverse Coordinates" ("Mode")
            n164 = call "Coordinate_rotation.vi"("Roll-Pitch-Yaw"=w568, "Input Position"=w567, "Mode"=w569) -> ("Output Position"=w565:sgl[])  [unwired: 2 in, 1 out]
            n165 = call "Coordinate_rotation.vi"("Roll-Pitch-Yaw"=w568, "Input Position"=w564, "Mode"=w569) -> ("Output Position"=w566:sgl[])  [unwired: 2 in, 1 out]
          }
        }
        n166 = call "Check_with_Jump_PN.vi"("Current position"=w522, "Traverse Name"=w530, "Simulate/Run"=w537, "New Position"=w524, "Traverse Active Parts"=cluster{"X":bool, "XY":bool, "XYZ":bool} {"X"=FALSE, "XY"=TRUE, "XYZ"=FALSE}, "Model       Roll      Pitch       Yaw (deg)"=w531) -> ("Error Comments"=w519:string, "Steps"=w521:sgl[][])  [unwired: 8 in]
        n167 = Empty String/Path?(string/path=w519) -> (empty?=w520:bool)
        n168 = case shown="True" w520 {
          tunnel: w522 -> [_ w550]
          tunnel: w521 -> [w541 w549]
          tunnel: [w541 w547] -> w533
          tunnel: w531 -> [_ w546]
          tunnel: [w542 w545] -> w539
          tunnel: w519 -> [w542 _]
          tunnel: w530 -> [_ w544]
          tunnel: w537 -> [_ w543]
          frame False {
          }
          frame True {
            n169 = for {
              shift-right: [w556] -> _
              shift-left: w550 -> [w561]
              tunnel: w549 -> [w556] mode=indexing
              shift-right: [w557] -> w547
              shift-left: sgl[][] [] -> [w558]
              tunnel: w546 -> [w555]
              tunnel: [w554] -> w545
              tunnel: w544 -> [w552]
              tunnel: w543 -> [w551]
              stop <- w553 continue-if-true
              n170 = call "Check_with_Jump_PN.vi"("Current position"=w561, "Traverse Name"=w552, "Simulate/Run"=w551, "New Position"=w556, "Traverse Active Parts"=cluster{"X":bool, "XY":bool, "XYZ":bool} {"X"=TRUE, "XY"=FALSE, "XYZ"=TRUE}, "Model       Roll      Pitch       Yaw (deg)"=w555) -> ("Error Comments"=w554:string, "Steps"=w559:sgl[][])  [unwired: 8 in]
              n171 = Empty String/Path?(string/path=w554) -> (empty?=w553:bool)
              n172 = Build Array (concatenate)(w558, w559) -> (w557:sgl[][])
            }
          }
        }
        n173 = Empty String/Path?(string/path=w539) -> (empty?=w528:bool)
        n174 = case shown="\"Don't Home\"" w534 {
          tunnel: w533 -> [w574 w581 w589 w597 w605 w613 w621]
          tunnel: [w574 w580 w588 w596 w604 w612 w620] -> w529
          tunnel: w532 -> [_ w575 w583 w591 w599 w607 w615]
          frame "Don't Home" {
          }
          frame "Home  +X" {
            n175 = for {
              tunnel: [w582] -> w579
              tunnel: w581 -> [w582] mode=indexing
            }
            n176 = Multiply(x=sgl[] [2.0, 0.0, 0.0] ("y"), y=w575) -> (x*y=w576:sgl[])
            n177 = Add(x=w579, y=w576) -> (x+y=w578:sgl[])
            n178 = Build Array (concatenate)(w581, w578) -> (w580:sgl[][])
          }
          frame "Home  -X" {
            n179 = for {
              tunnel: [w590] -> w587
              tunnel: w589 -> [w590] mode=indexing
            }
            n180 = Multiply(x=sgl[] [-2.0, 0.0, 0.0] ("y"), y=w583) -> (x*y=w584:sgl[])
            n181 = Add(x=w587, y=w584) -> (x+y=w586:sgl[])
            n182 = Build Array (concatenate)(w589, w586) -> (w588:sgl[][])
          }
          frame "Home  +Y" {
            n183 = for {
              tunnel: [w598] -> w595
              tunnel: w597 -> [w598] mode=indexing
            }
            n184 = Multiply(x=sgl[] [0.0, 2.0, 0.0] ("y"), y=w591) -> (x*y=w592:sgl[])
            n185 = Add(x=w595, y=w592) -> (x+y=w594:sgl[])
            n186 = Build Array (concatenate)(w597, w594) -> (w596:sgl[][])
          }
          frame "Home  -Y" {
            n187 = for {
              tunnel: [w606] -> w603
              tunnel: w605 -> [w606] mode=indexing
            }
            n188 = Multiply(x=sgl[] [0.0, -2.0, 0.0] ("y"), y=w599) -> (x*y=w600:sgl[])
            n189 = Add(x=w603, y=w600) -> (x+y=w602:sgl[])
            n190 = Build Array (concatenate)(w605, w602) -> (w604:sgl[][])
          }
          frame "Home  +Z" {
            n191 = for {
              tunnel: [w614] -> w611
              tunnel: w613 -> [w614] mode=indexing
            }
            n192 = Multiply(x=sgl[] [0.0, 0.0, 2.0] ("y"), y=w607) -> (x*y=w608:sgl[])
            n193 = Add(x=w611, y=w608) -> (x+y=w610:sgl[])
            n194 = Build Array (concatenate)(w613, w610) -> (w612:sgl[][])
          }
          frame "Home  -Z" {
            n195 = for {
              tunnel: [w622] -> w619
              tunnel: w621 -> [w622] mode=indexing
            }
            n196 = Multiply(x=sgl[] [0.0, 0.0, -2.0] ("y"), y=w615) -> (x*y=w616:sgl[])
            n197 = Add(x=w619, y=w616) -> (x+y=w618:sgl[])
            n198 = Build Array (concatenate)(w621, w618) -> (w620:sgl[][])
          }
        }
        n199 = case shown="True" w528 {
          tunnel: ["Route Error" "Perform Trav 2 Trav Check"] -> w527
          tunnel: [w570 TRUE] -> w526
          tunnel: w525 -> [w570 _]
          frame False {
          }
          frame True {
          }
        }
      }
      frame "Perform Trav 2 Trav Check" {
        n200 = case shown="\"Work in Tunnel Coordinates\"" w632 {
          tunnel: w626 -> [w645 w648]
          tunnel: [w645 w647] -> w631
          tunnel: w633 -> [_ w646]
          frame "Work in Tunnel Coordinates" {
          }
          frame "Work in Model Coordinates" {
            n201 = call "Coordinate_rotation.vi"("Roll-Pitch-Yaw"=w646, "Input Position"=w648, "Mode"=T7."To Traverse Coordinates") -> ("Output Position"=w647:sgl[])  [unwired: 2 in, 1 out]
          }
        }
        n202 = for {
          tunnel: w634 -> [w659]
          tunnel: w623 -> [w655] mode=indexing
          tunnel: w640 -> [w658]
          tunnel: [w657] -> w639
          tunnel: [w656] -> w638
          shift-right: [w655] -> _
          shift-left: w631 -> [w654]
          stop <- w656 continue-if-true
          n203 = call "Traverse_to_Traverse_Collision.vi"("Current Position  (Tun Coord)"=w654, "Traverse Name"=w659, "Simulate/Run"=w658, "New Position (Tun Coord)"=w655) -> ("Error String"=w657:string)  [unwired: 7 in]
          n204 = Empty String/Path?(string/path=w657) -> (empty?=w656:bool)
        }
        n205 = Empty String/Path?(string/path=w625) -> (empty?=w624:bool)
        n206 = case shown="True" w638 {
          tunnel: ["Route Error" "Display Traverse Views" ("f")] -> w637
          tunnel: [w650 TRUE] -> w636
          tunnel: w635 -> [w650 _]
          frame False {
          }
          frame True {
          }
        }
        n207 = Concatenate Strings(w625, w639) -> (w630:string)
        n208 = case shown="True" w624 {
          tunnel: w623 -> [_ w642]
          frame False {
          }
          frame True {
            "Valid Steps before Trav to Trav (Tun Cord)" <- w642
          }
        }
        n209 = Empty String/Path?(string/path=w630) -> (empty?=w629:bool)
        n210 = case shown="False" w629 {
          tunnel: [w643 w644] -> w628
          tunnel: w627 -> [_ w644]
          tunnel: w626 -> [w643 _]
          frame False {
          }
          frame True {
          }
        }
      }
      frame "Route Error" {
        n211 = global read "Trav_pos_global.vi" "Current Row"() -> (w665:T11)
        n212 = global read "Extra_Commands_Global.vi" "Suppress Route Check Errors"() -> (w663:string)
        n213 = Unbundle By Name(w665) -> ("Extra Commands"=w664:string)
        n214 = call "Extra_Commands.vi"("String to Search"=w664, "Command"=w663) -> ("Command Found"=w662:bool)  [unwired: 1 in, 4 out]
        n215 = Concatenate Strings("Route Checking Error\n" ("string"), w673) -> (w661:string)
        n216 = case shown="False" w668 {
          tunnel: w672 -> [w697 _]
          tunnel: w670 -> [w698 _]
          tunnel: w669 -> [w682 _]
          tunnel: [w679 "Display Traverse Views"] -> w666
          tunnel: w665 -> [w690 _]
          tunnel: w662 -> [w688 _]
          tunnel: w661 -> [w685 _]
          tunnel: w660 -> [w681 _]
          frame False {
            n217 = Unbundle By Name(w690) -> ("Row No"=w691:i32)
            n218 = case shown="\"Work in Tunnel Coordinates\"" w698 {
              tunnel: [w700 w703] -> w696
              tunnel: w697 -> [w701 w703]
              tunnel: w682 -> [w699 _]
              frame "Work in Tunnel Coordinates" {
                n219 = call "Coordinate_rotation.vi"("Roll-Pitch-Yaw"=w699, "Input Position"=w701, "Mode"=T7."To User Coordinates") -> ("Output Position"=w700:sgl[])  [unwired: 2 in, 1 out]
              }
              frame "Work in Model Coordinates" {
              }
            }
            n220 = Number To Decimal String(number=w691) -> (decimal integer string=w684:string)  [unwired: 1 in]
            n221 = Array Subset(array=w696, length=3) -> (w694:sgl[])  [unwired: 1 in]
            n222 = Select(t="Suppressed", s=w688, f="") -> (s? t:f=w683:string)
            n223 = Number To Fractional String(number=w694, precision (6)=i16 0) -> (F-format string=w692:string[])  [unwired: 2 in]
            n224 = Select(t="Save Position Information", s=w681, f="End") -> (s? t:f=w679:string)
            n225 = Build Array (concatenate)(w684, w692, w683, w685) -> (w689:string[])
            n226 = call "MultiRun Status.vi"("Input Array"=w689) -> ()  [unwired: 1 out]
          }
          frame True {
          }
        }
      }
      frame "Save Position Information" {
        n227 = case shown="\"Work in Model Coordinates\"" w709 {
          tunnel: [w716 w718] -> w706
          tunnel: w707 -> [w716 w719]
          tunnel: w708 -> [_ w717]
          frame "Work in Tunnel Coordinates" {
          }
          frame "Work in Model Coordinates" {
            n228 = call "Coordinate_rotation.vi"("Roll-Pitch-Yaw"=w717, "Input Position"=w719, "Mode"=T7."To Traverse Coordinates") -> ("Output Position"=w718:sgl[])  [unwired: 2 in, 1 out]
          }
        }
        n229 = call "Save_Position_Checking.vi"("Traverse Name"=w705, "Error String"=w710, "Model       Roll      Pitch       Yaw (deg)"=w708, "Position"=w706) -> ()  [unwired: 2 in]
      }
      frame "Display Traverse Views" {
        n230 = global read "Route_mapping_global.vi" "Display Mode"() -> (w737:T8)
        n231 = Equal?(x=w732, y=User_Specific_mode."Check VI only" ("Simulate/Run")) -> (x = y?=w731:bool)
        n232 = Empty String/Path?(string/path=w735) -> (empty?=w722:bool)
        n233 = Equal?(x=w737, y=Route_Display_Mode."Display View Always" ("Display Mode")) -> (x = y?=w734:bool)
        n234 = Not(x=w722) -> (.not. x?=w728:bool)
        n235 = Or(x=w734, y=w728) -> (x .or. y?=w730:bool)
        n236 = And(x=w731, y=w730) -> (x .and. y?=w729:bool)
        n237 = case shown="True" w729 {
          tunnel: w739 -> [_ w753]
          tunnel: w738 -> [_ w752]
          tunnel: w735 -> [_ w749]
          tunnel: w722 -> [_ w747]
          frame False {
          }
          frame True {
            n238 = Not(x=w747) -> (.not. x?=w748:bool)
            n239 = call "MultiRun Status.vi"() -> ("Table Control"=w744:string[][])  [unwired: 1 in]
            n240 = Index Array(array=w744, index (row)=0) -> (element=w745:string[])  [unwired: 1 in]
            n241 = for {
              tunnel: w753 -> [w758] mode=indexing
              tunnel: w752 -> [w764]
              tunnel: "Currently on Point" -> [w763]
              tunnel: "Row Number" -> [w762]
              tunnel: w749 -> [w761]
              tunnel: w748 -> [w759]
              tunnel: w745 -> [w756]
              n242 = Number To Fractional String(number=w758, precision (6)=i16 1) -> (F-format string=w755:string[])  [unwired: 2 in]
              n243 = Build Array(w756, w755) -> (w754:string[][])
              n244 = call "Display_Trav_Views.vi"("Probe Positions"=w754, "Traverse Name"=w764, "Currently on point"=w763, "Open Front Panel"=TRUE, "Error Comments"=w761, "Crash?"=w759, "Row Number"=w762) -> ()  [unwired: 4 out]
            }
          }
        }
        n245 = case shown="\"Run VI\"" w732 {
          tunnel: ["Calculate Move Time" "Execute case"] -> w723
          tunnel: w722 -> [_ _]
          frame "Check VI only" {
          }
          frame "Run VI" {
          }
        }
        n246 = Select(t=w723, s=w722, f="End") -> (s? t:f=w721:string)
      }
      frame "Calculate Move Time" {
        n247 = local read "Start Position"() -> (w768:sgl[])
        n248 = call "Calculate_3D_Move_Time.vi"("Model:    Roll        Pitch         Yaw  (deg)"=w771, "Work in Tunnel Coordinates"=w772, "Backlash?"=w766, "Traverse Setup"=w765, "Positions"=w769, "Start Position"=w768) -> ("Time (s)"=→"Move Time (s)":sgl)  [unwired: 5 in]
      }
      frame "Execute case" {
        n249 = Array Size(array=w791) -> (size(s)=w792:i32[])
        n250 = Index Array(array=w792) -> (element=w790:i32)  [unwired: 1 in]
        n251 = global read "Trav_pos_global.vi" "Fast Plotting?"() -> (w781:bool)
        n252 = Decrement(x=w790) -> (x-1=w789:i32)
        n253 = Select(t=TRUE, s=w786, f=w783) -> (s? t:f=w784:bool)
        n254 = for {
          tunnel: w800 -> [w824]
          tunnel: w791 -> [w827] mode=indexing
          tunnel: w793 -> [w826]
          tunnel: w799 -> [w822]
          tunnel: [w828] -> w798
          tunnel: [w823] -> w787
          tunnel: w795 -> [w825]
          tunnel: w789 -> [w819]
          tunnel: w788 -> [w814]
          tunnel: w780 -> [w817]
          tunnel: w784 -> [w813]
          tunnel: w779 -> [w812]
          tunnel: w782 -> [w810]
          tunnel: w781 -> [w809]
          tunnel: w778 -> [w802]
          i -> [w818]
          stop <- w821 continue-if-true
          w815 = Home."Don't Home" ("Home")
          n255 = Not Equal?(x=w814, y=w815) -> (x != y?=w816:bool)
          n256 = Subtract(x=w819, y=w818) -> (x-y=w811:i32)
          n257 = Equal To 0?(x=w811) -> (x = 0?=w803:bool)
          n258 = case shown="1" w811 {
            tunnel: [w836 w840 w844] -> w806
            tunnel: [w834 w839 w841] -> w820
            tunnel: w817 -> [w838 _ w846]
            tunnel: [w833 w840 FALSE ("f")] -> w808
            tunnel: w816 -> [w835 _ w842]
            tunnel: w815 -> [_ w839 w841]
            tunnel: w814 -> [w834 _ _]
            tunnel: w813 -> [w833 _ _]
            frame 0 {
              n259 = Select(t=FALSE, s=w835, f=w838) -> (s? t:f=w836:bool)
            }
            frame Default {
              w840 = FALSE ("f")
            }
            frame 1 {
              n260 = Select(t=w846, s=w842, f=FALSE) -> (s? t:f=w844:bool)
            }
          }
          n261 = case shown="False" w809 {
            tunnel: w808 -> [w831 _]
            tunnel: [w831 w832] -> w807
            tunnel: w806 -> [w830 _]
            tunnel: [w830 w832] -> w805
            tunnel: [w829 w832] -> w804
            tunnel: w803 -> [w829 _]
            frame False {
            }
            frame True {
              w832 = FALSE
            }
          }
          n262 = call "TraverseControl_High.vi"("Mode"=w826, "Route Checking?"=w825, "Home"=w820, "Traverse Name"=w824, "Extra command String"=w812, "Work in Tunnel Coordinates"=w810, "Model       Roll      Pitch       Yaw (deg)"=w822, "Final iteration of 3D_Trav Loop"=w804, "Position input XYZ Always Tunnel"=w827, "Last Part of Move?"=w807, "Speed Factor"=w802, "Backlash Compensation?"=w805) -> ("Position Output XYZ"=w828:sgl[], "Error String"=w823:string)  [unwired: 1 in, 1 out]
          n263 = Empty String/Path?(string/path=w823) -> (empty?=w821:bool)
        }
        n264 = case shown="\"Work in Model Coordinates\"" w782 {
          tunnel: w798 -> [w847 w850]
          tunnel: [w847 w849] -> w797
          tunnel: w799 -> [_ w848]
          frame "Work in Tunnel Coordinates" {
          }
          frame "Work in Model Coordinates" {
            n265 = call "Coordinate_rotation.vi"("Roll-Pitch-Yaw"=w848, "Input Position"=w850, "Mode"=T7."To User Coordinates") -> ("Output Position"=w849:sgl[])  [unwired: 2 in, 1 out]
          }
        }
      }
      frame "Update Position Globals" {
        n266 = case shown="\"Check VI only\"" w856 {
          tunnel: w855 -> [w866 _]
          tunnel: w854 -> [w865 _]
          tunnel: w853 -> [w864 _]
          tunnel: w852 -> [w863 _]
          frame "Check VI only" {
            n267 = stacked-sequence {
              seq-local: [w867 _] -> [_ w879]
              tunnel: w866 -> [_ w882]
              tunnel: w865 -> [w868 _]
              tunnel: w864 -> [w870 _]
              tunnel: w863 -> [w869 _]
              frame #0 {
                n268 = case shown="\"Work in Model Coordinates\"" w870 {
                  tunnel: w868 -> [w871 w874]
                  tunnel: [w871 w873] -> w867
                  tunnel: w869 -> [_ w872]
                  frame "Work in Tunnel Coordinates" {
                  }
                  frame "Work in Model Coordinates" {
                    n269 = call "Coordinate_rotation.vi"("Roll-Pitch-Yaw"=w872, "Input Position"=w874, "Mode"=T7."To Traverse Coordinates") -> ("Output Position"=w873:sgl[])  [unwired: 2 in, 1 out]
                  }
                }
              }
              frame #1 {
                n270 = global read "Trav_pos_global.vi" "Route checking Chs"() -> (w881:string[])
                n271 = global read "Trav_pos_global.vi" "ADAM Positions Ch names"() -> (w880:string[])
                n272 = for {
                  tunnel: w882 -> [w893]
                  tunnel: w881 -> [w892]
                  tunnel: w880 -> [w889]
                  tunnel: w879 -> [w888] mode=indexing
                  tunnel: [w887] -> w876 mode=indexing if=w883
                  tunnel: [w886] -> w877 mode=indexing if=w883
                  i -> [w895]
                  n273 = Format Into String(format string="%d", initial string=w893, w895) -> (resulting string=w891:string)  [unwired: 1 in, 1 out]
                  n274 = Search 1D Array(1D array=w892, element=w891) -> (index of element=w890:i32)  [unwired: 1 in]
                  n275 = Index Array(array=w889, index=w890) -> (element=w886:string)
                  n276 = Empty String/Path?(string/path=w886) -> (empty?=w884:bool)
                  n277 = Not(x=w884) -> (.not. x?=w883:bool)
                  n278 = Number To Fractional String(number=w888, precision (6)=i16 4) -> (F-format string=w887:string)  [unwired: 2 in]
                }
                n279 = call "Read_Write_Local_table_Quick.vi"("Mode"=Quick_local_ADAM_Table."Write Global", "String Values In"=w876, "Ch names In"=w877) -> ()  [unwired: 3 out]
              }
            }
          }
          frame "Run VI" {
          }
        }
        n280 = global write "Trav_pos_global.vi" "Traverse position"(w854) -> ()
        n281 = global write "Trav_pos_global.vi" "Live Position"(w854) -> ()
      }
      frame "Tidy up" {
        w896 = User_Specific_mode."Run VI" ("Simulate/Run")
        n282 = case shown="\"Move traverse\"" w901 {
          tunnel: w907 -> [w921 w988]
          tunnel: w906 -> [w922 w987]
          tunnel: w902 -> [w920 _]
          tunnel: [w919 w987] -> w905
          tunnel: w900 -> [w915 _]
          tunnel: w899 -> [w918 _]
          tunnel: w898 -> [w914 _]
          tunnel: w897 -> [w917 _]
          tunnel: w896 -> [w916 _]
          frame "Move traverse" {
            n283 = Equal?(x=w914, y=w916) -> (x = y?=w913:bool)
            n284 = And(x=w917, y=w913) -> (x .and. y?=w912:bool)
            n285 = case shown="False" w912 {
              tunnel: w922 -> [w927 w964]
              tunnel: w921 -> [w926 w967]
              tunnel: w920 -> [w925 _]
              tunnel: [w924 w962] -> w919
              tunnel: w918 -> [_ w961]
              tunnel: w915 -> [_ w958]
              frame False {
                n286 = Empty String/Path?(string/path=w927) -> (empty?=w923:bool)
                n287 = case shown="True" w923 {
                  tunnel: w926 -> [_ w932]
                  tunnel: w925 -> [_ w931]
                  tunnel: w927 -> [w928 w930]
                  tunnel: [w928 w929] -> w924
                  frame False {
                  }
                  frame True {
                    n288 = for {
                      tunnel: w932 -> [w935] mode=indexing
                      tunnel: w931 -> [w936] mode=indexing
                      shift-right: [w933] -> w929
                      shift-left: w930 -> [w934]
                      i -> [w939]
                      w941 = 10.0  # ±
                      n289 = case shown="0, Default" w939 {
                        tunnel: ["X" "Y" "Z"] -> w937
                        frame 0, Default {
                        }
                        frame 1 {
                        }
                        frame 2 {
                        }
                      }
                      n290 = call "In_Range_check.vi"("±"=w941, "Mode"=In_Range."±", "Value"=w936, "Setpoint"=w935) -> ("In Range"=w938:bool)  [unwired: 1 in, 2 out]
                      n291 = case shown="False" w938 {
                        tunnel: w937 -> [w948 _]
                        tunnel: w936 -> [w947 _]
                        tunnel: w935 -> [w946 _]
                        tunnel: w934 -> [w943 w949]
                        tunnel: [w944 w949] -> w933
                        frame False {
                          n292 = Format Into String(format string="For %s Axis Dem Pos = %.1f Achieved Pos = %.1f mm" ("Format String"), w948, w947, w946) -> (resulting string=w942:string)  [unwired: 2 in, 1 out]
                          n293 = Concatenate Strings(w943, w942) -> (w944:string)
                        }
                        frame True {
                        }
                      }
                    }
                  }
                }
              }
              frame True {
                n294 = local read "Position"() -> (w953:sgl[])
                n295 = case shown="\"Home  -X\"" w958 {
                  tunnel: [0 ("index") 0 ("index") 0 ("index") 1 ("index") 1 ("index") 2 ("index") 2 ("index")] -> w957
                  tunnel: ["-X" "+X" "-X" "+Y" "-Y" "+Z" "-Z"] -> w956
                  frame "Don't Home" {
                  }
                  frame "Home  +X" {
                  }
                  frame "Home  -X" {
                  }
                  frame "Home  +Y" {
                  }
                  frame "Home  -Y" {
                  }
                  frame "Home  +Z" {
                  }
                  frame "Home  -Z" {
                  }
                }
                n296 = Index Array(array=w967, index=w957) -> (element=w955:sgl)
                n297 = Index Array(array=w953, index=w957) -> (element=w954:sgl)
                n298 = Subtract(x=w955, y=w954) -> (x-y=w960:sgl)
                n299 = Multiply(x=0.995, y=w961) -> (x*y=w965:dbl)
                n300 = Absolute Value(x=w960) -> (abs(x)=w959:sgl)
                n301 = Less?(x=w959, y=w965) -> (x < y?=w963:bool)
                n302 = case shown="False" w963 {
                  tunnel: w964 -> [w985 w986]
                  tunnel: [w984 w986] -> w962
                  tunnel: w956 -> [w982 _]
                  frame False {
                    n303 = Concatenate Strings(w985, w982, " home has not been found.") -> (w984:string)
                  }
                  frame True {
                  }
                }
              }
            }
          }
          frame "Read traverse position", Default {
            n304 = local write "Position"(w988) -> ()
          }
        }
        n305 = local write "Currently on Point"(-1 ("Row Number")) -> ()
        n306 = local write "Simulate/Run"(w896) -> ()
      }
      frame "End" {
        n307 = case shown="Default" w997 {
          frame "Move traverse" {
          }
          frame Default {
            n308 = local write "Mode"(Trav_mode."Move traverse" ("Mode")) -> ()
            n309 = local write "Position Offset"(sgl[] [0.0, 0.0, 0.0] ("Position Offset")) -> ()
          }
        }
        n310 = local write "Route Checking?"(TRUE ("Route Checking?")) -> ()
        n311 = case shown="\"Work in Tunnel Coordinates\"" w1001 {
          tunnel: w1000 -> [w1007 w1010]
          tunnel: [w1007 w1009] -> w991
          tunnel: w999 -> [_ w1008]
          frame "Work in Tunnel Coordinates" {
          }
          frame "Work in Model Coordinates" {
            n312 = call "Coordinate_rotation.vi"("Roll-Pitch-Yaw"=w1008, "Input Position"=w1010, "Mode"=T7."To Traverse Coordinates") -> ("Output Position"=w1009:sgl[])  [unwired: 2 in, 1 out]
          }
        }
        n313 = global read "Trav_pos_global.vi" "Trav_Coordinates Current Pos dx;dy;dz"() -> (w990:sgl[])
        n314 = local write "Home"(Home."Don't Home" ("Home")) -> ()
        n315 = Empty String/Path?(string/path=w994) -> (empty?=w996:bool)
        n316 = case shown="False" w996 {
          tunnel: [w1014 w1016] -> w995
          tunnel: w994 -> [w1013 w1016]
          tunnel: w993 -> [w1012 _]
          frame False {
            n317 = Format Into String(format string="%s Traverse Error\n%s", w1012, w1013) -> (resulting string=w1014:string)  [unwired: 2 in, 1 out]
          }
          frame True {
          }
        }
        n318 = call "Read-Write_Check_Pos.vi"("Simulate/Run"=w989, "!Offset Position by dx;dy;dz  Input"=w990, "Position input"=w991, "Mode"=enum16{"Read", "Write"}."Write", "Traverse Name"=w993) -> ()  [unwired: 2 in, 3 out]
      }
    }
  }
  "Trav Position achieved" <- w19
  "Error String" <- w22
